vi "download_calibration_rm_vlc.vi"(9 "port":u16, 10 "host":string, 11 "path in":path=path "hl2ss_ulm.dll") -> (1 "error":bool, 2 "calibration":T1, 3 "path out":path)   [LabVIEW 2023]
panel:
  in  "calibration":T1
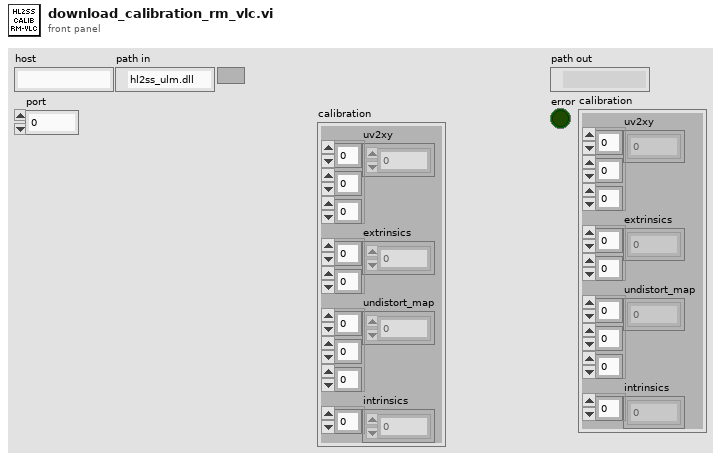
[diagram p1: front panel]
types:
  T1 = cluster{"uv2xy":sgl[][][], "extrinsics":sgl[][], "undistort_map":sgl[][][], "intrinsics":sgl[]}
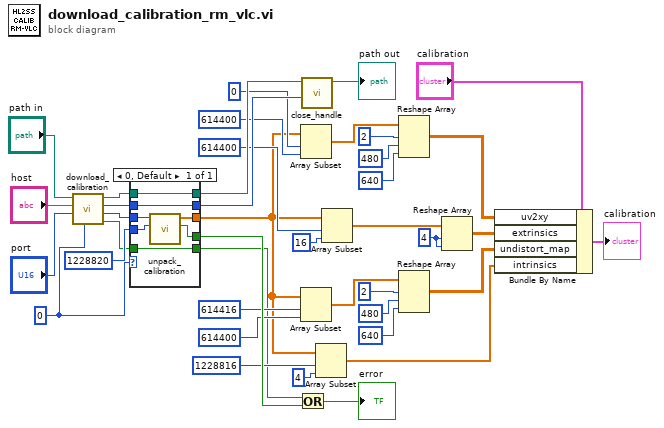
[diagram p0: block diagram]
diagram:
  w10 = 4 ("dimension size")
  w37 = u64 0 ("configuration")
  n1 = call "download_calibration.vi"("configuration"=w37, "port"="port", "host"="host", "path in"="path in") -> ("error"=w1:bool, "calibration"=w35:u64, "calibration_handle"=w33:u64, "path out"=w34:path)  [unwired: 4 in]
  n2 = case shown="0, Default" w37 {
    tunnel: 1228820 ("element_count") -> [w47]
    tunnel: w35 -> [w46]
    tunnel: w34 -> [w45]
    tunnel: w33 -> [w44]
    tunnel: [w45] -> w32
    tunnel: [w44] -> w31
    tunnel: [w43] -> w22
    tunnel: [w42] -> w30
    tunnel: [w41] -> w2
    tunnel: w1 -> [w41]
    frame 0, Default {
      n3 = call "unpack_calibration.vi"("element_count"=w47, "calibration"=w46) -> ("error"=w42:bool, "calibration"=w43:sgl[])  [unwired: 8 in]
    }
  }
  n4 = Or(x=w2, y=w30) -> (x .or. y?=→"error":bool)
  n5 = Array Subset(array=w22, index=0, length=614400) -> (w19:sgl[])
  n6 = Array Subset(array=w22, index=614416, length=614400) -> (w18:sgl[])
  n7 = call "close_handle.vi"("handle"=w31, "path in"=w32) -> ("path out"=→"path out":path)  [unwired: 9 in]
  n8 = Array Subset(array=w22, index=1228816, length=4) -> (w5:sgl[])
  n9 = Array Subset(array=w22, index=614400, length=16) -> (w17:sgl[])
  n10 = Reshape Array(w19, 2 ("dimension size"), 480 ("dimension size"), 640 ("dimension size")) -> (w8:sgl[][][])
  n11 = Reshape Array(w18, 2 ("dimension size"), 480 ("dimension size"), 640 ("dimension size")) -> (w6:sgl[][][])
  n12 = Reshape Array(w17, w10, w10) -> (w7:sgl[][])
  n13 = Bundle By Name(cluster="calibration", "uv2xy"=w8, "extrinsics"=w7, "undistort_map"=w6, "intrinsics"=w5) -> (→"calibration":T1)
